vi "Interface connect.vi"(8 "error in (no error)":errorcluster, 11 "TCP interface in":refnum<class "TCP Interface.lvclass">) -> (0 "error out":errorcluster, 3 "TCP interface out":refnum<class "TCP Interface.lvclass">)   [LabVIEW 2021, in "TCP Interface.lvclass"]
doc: "Opens a TCP connection to the address and port stored in the class."
uses:
  TCP Interface.lvclass
  TCP Interface.lvclass/TCP Interface.ctl
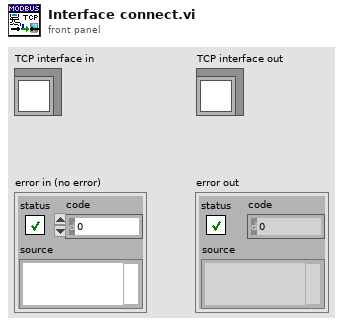
[diagram p1: front panel]
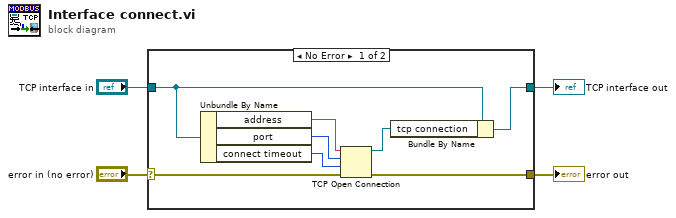
[diagram p0: block diagram]
diagram:
  n1 = case shown="No Error" "error in (no error)" {
    selector: "error in (no error)" -> [w6 w13]
    tunnel: [w10 w13] -> w4
    tunnel: "TCP interface in" -> [w9 w14]
    tunnel: [w7 w14] -> w2
    frame No Error {
      n2 = Unbundle By Name(w9) -> ("address"=w12:string, "port"=w11:u16, "connect timeout"=w5:i32)
      n3 = TCP Open Connection(address=w12, remote port or service name=w11, timeout ms (60000)=w5, error in (no error)=w6) -> (connection ID=w8:refnum<k5>, error out=w10:errorcluster)  [unwired: 1 in]
      n4 = Bundle By Name(cluster=w9, "tcp connection"=w8) -> (w7:refnum<class "TCP Interface.lvclass">)
    }
    frame Error {
    }
  }
  "error out" <- w4
  "TCP interface out" <- w2
